vi "StatIntialse.vi"(0 "Init cluster 2":T1, 1 "Set Stability":T2(ring)=enum."Standard", 2 "Default\n Filter":T3(ring)=enum."10 kHz", 3 "error in (no error)":errorcluster, 4 "Default\nCurrent range":T4(ring)=enum."10 mA") -> (7 "Init cluster":T1, 10 "error out":errorcluster)   [LabVIEW 2020]
uses:
  Labview/IVIUM/IVIUM_remdriver.lvlib
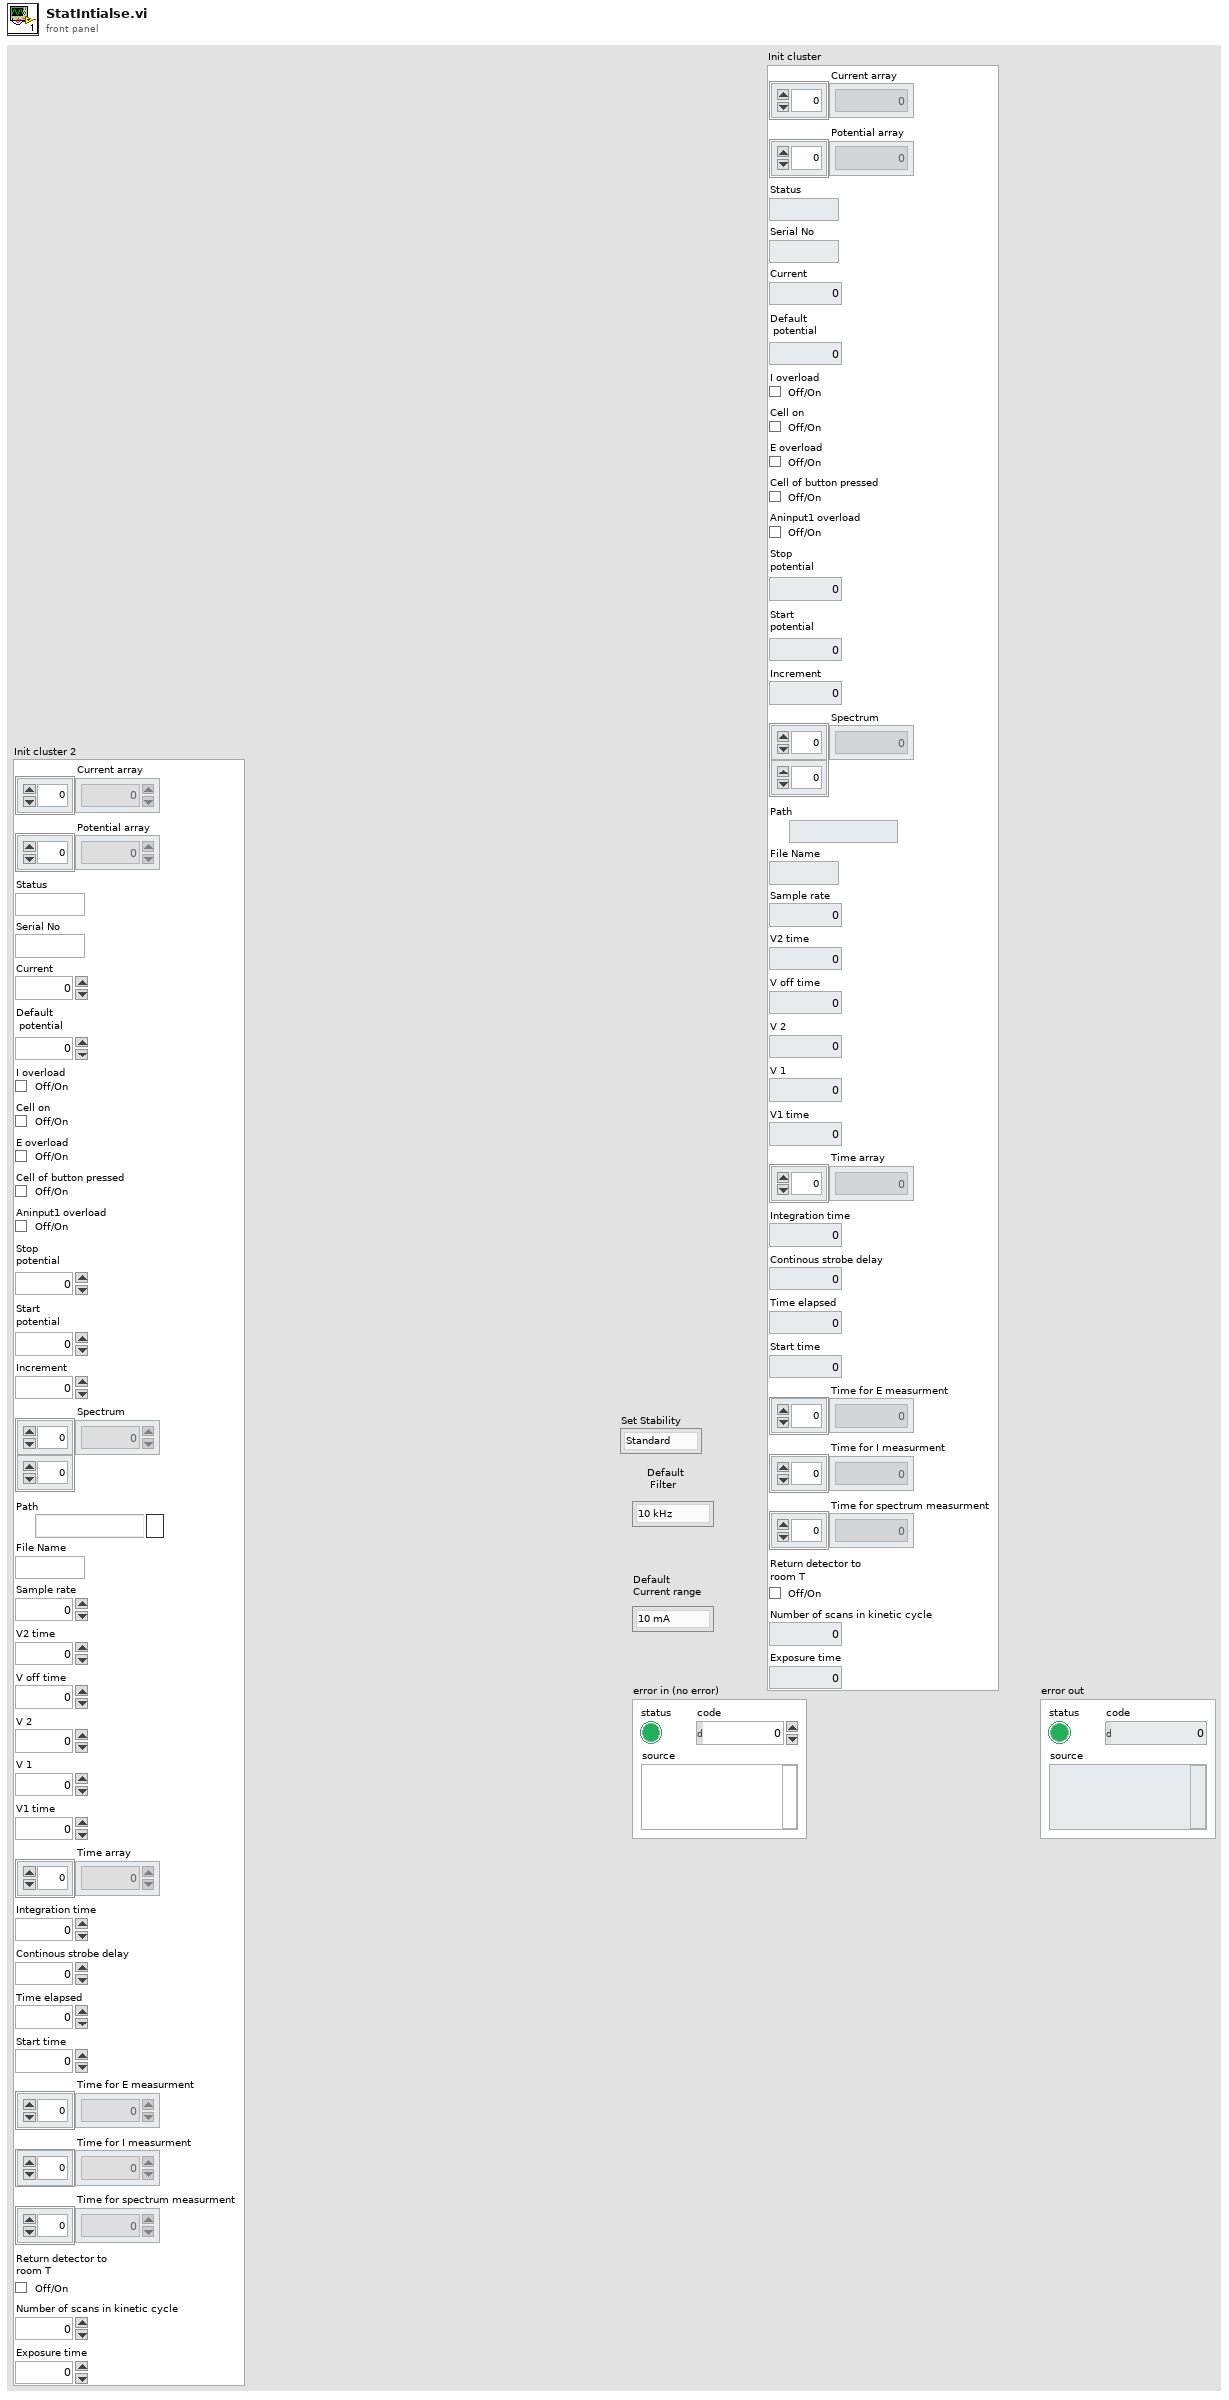
[diagram p1: front panel]
types:
  T1 = cluster{"Current array":dbl[], "Potential array":dbl[], "Status":string, "Serial No":string, "Current":dbl, "Default\n potential":dbl, "I overload":bool, "Cell on":bool, "E overload":bool, "Cell of button pressed":bool, "Aninput1 overload":bool, "Stop \npotential":dbl, "Start \npotential":dbl, "Increment":dbl, "Spectrum":dbl[][], "Path":path, "File Name":string, "Sample rate":dbl, "V2 time":dbl, "V off time":dbl, "V 2":dbl, "V 1":dbl, "V1 time":dbl, "Time array":dbl[], "Integration time":i32, "Continous strobe delay":i32, "Time elapsed ":i32, "Start time":i32, "Time for E measurment":i32[], "Time for I measurment ":i32[], "Time for spectrum measurment":i32[], "Return detector to \nroom T":bool, "Number of scans in kinetic cycle":i32, "Exposure time":i32}
  T2 = enum16{"High Speed", "Standard", "High Stability"}
  T3 = enum16{"1 MHz", "100 kHz", "10 kHz", "1 kHz", "10 Hz"}
  T4 = enum16{"10 A", "1 A", "100 mA", "10 mA", "1 mA", "100 uA", "10 uA", "1 uA", "100 nA", "10 nA", "1 nA", "100 pA", "10 pA", "1 pA"}
  T5 = enum16{"off", "EStat4EL", "EStat2EL", "EStatDummy1", "EStatDummy2", "EStatDummy3", "EStatDummy4", "IStat4EL", "IStat2EL", "IStatDummy", "BiStat4EL", "BiStat2EL"}
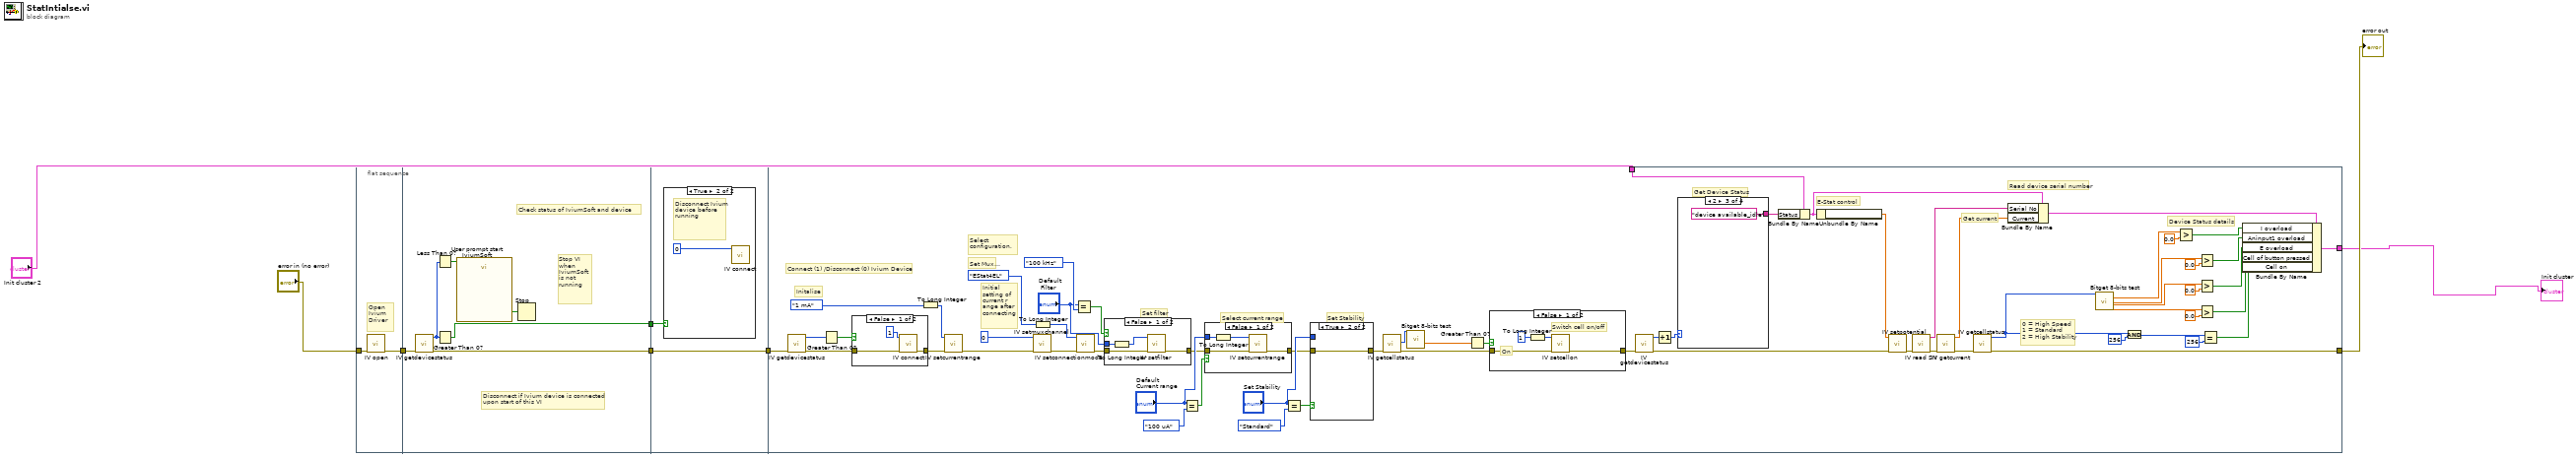
[diagram p0: block diagram]
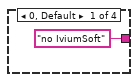
[diagram p5: hidden frame]
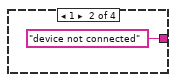
[diagram p6: hidden frame]
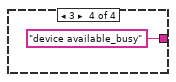
[diagram p7: hidden frame]
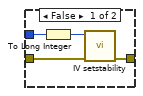
[diagram p8: hidden frame]
diagram:
  n1 = flat-sequence {
    tunnel: [w10] -> w7
    tunnel: "error in (no error)" -> [w9]
    tunnel: w7 -> [w13]
    tunnel: [w12] -> w5
    tunnel: [w11] -> w3
    tunnel: w5 -> [w18]
    tunnel: [w18] -> w4
    tunnel: w3 -> [w17]
    tunnel: "Init cluster 2" -> [w31]
    tunnel: [w45] -> w8
    tunnel: w4 -> [w22]
    tunnel: [w20] -> w1
    frame #0 {
      # "Open Ivium Driver"
      n2 = call "IV open.vi"("error in (no error)"=w9) -> ("error out"=w10:errorcluster)  [unwired: 9 in, 1 out]
    }
    frame #1 {
      # "Check status of IviumSoft and device"
      # "Stop VI when IviumSoft is not running"
      # "Disconnect if Ivium device is connected \nupon start of this VI"
      n3 = call "IV getdevicestatus.vi"("error in (no error)"=w13) -> ("error out"=w12:errorcluster, "return type"=w16:i32)  [unwired: 9 in]
      n4 = Less Than 0?(x=w16) -> (x < 0?=w14:bool)
      n5 = Greater Than 0?(x=w16) -> (x > 0?=w11:bool)
      n6 = call "User prompt start IviumSoft.vi"("Enable"=w14) -> ("OK"=w15:bool)  [unwired: 17 in, 1 out]
      n7 = Stop(stop? (T)=w15) -> ()
    }
    frame #2 {
      n8 = case shown="True" w17 {
        frame False {
        }
        frame True {
          # "Disconnect Ivium device before running"
          n9 = call "IV connect.vi"("devconnect"=0) -> ()  [unwired: 8 in, 3 out]
        }
      }
    }
    frame #3 {
      # "Device Status details"
      # "Get current"
      # "Set Mux channel"
      # "0 = High Speed\n1 = Standard \n2 = High Stability"
      # "Set Stability"
      # "Set filter"
      # "E-Stat control"
      # "Get Device Status"
      # "Select current range"
      # "Select configuration,"
      # "Read device serial number"
      # "Initial setting of current r\nange after connecting"
      # "Connect (1) /Disconnect (0) Ivium Device"
      # "Initalise"
      n10 = call "IV getdevicestatus.vi"("error in (no error)"=w22) -> ("error out"=w42:errorcluster, "return type"=w44:i32)  [unwired: 9 in]
      n11 = Greater Than 0?(x=w44) -> (x > 0?=w43:bool)
      n12 = case shown="False" w43 {
        tunnel: [w84 w85] -> w41
        tunnel: w42 -> [w82 w85]
        frame False {
          n13 = call "IV connect.vi"("error in (no error)"=w82, "devconnect"=1) -> ("error out"=w84:errorcluster)  [unwired: 7 in, 2 out]
        }
        frame True {
        }
      }
      n14 = To Long Integer(number=T4."1 mA" ("Current range selector")) -> (32bit integer=w40:i32)
      n15 = call "IV setcurrentrange.vi"("error in (no error)"=w41, "value"=w40) -> ("error out"=w39:errorcluster)  [unwired: 7 in, 2 out]
      n16 = call "IV setmuxchannel.vi"("error in (no error)"=w39, "value"=0) -> ("error out"=w38:errorcluster)  [unwired: 7 in, 2 out]
      n17 = To Long Integer(number=T5."EStat4EL" ("Configuration")) -> (32bit integer=w37:i32)
      n18 = Equal?(x="Default\n Filter", y=T3."100 kHz" ("Set Filter")) -> (x = y?=w75:bool)
      n19 = call "IV setconnectionmode.vi"("error in (no error)"=w38, "value"=w37) -> ("error out"=w35:errorcluster)  [unwired: 7 in, 2 out]
      n20 = case shown="False" w75 {
        tunnel: "Default\n Filter" -> [w103 _]
        tunnel: [w101 w104] -> w36
        tunnel: w35 -> [w100 w104]
        frame False {
          n21 = To Long Integer(number=w103) -> (32bit integer=w102:i32)
          n22 = call "IV setfilter.vi"("error in (no error)"=w100, "value"=w102) -> ("error out"=w101:errorcluster)  [unwired: 7 in, 2 out]
        }
        frame True {
        }
      }
      n23 = Equal?(x="Default\nCurrent range", y=T4."100 uA") -> (x = y?=w79:bool)
      n24 = case shown="False" w79 {
        tunnel: "Default\nCurrent range" -> [w107 _]
        tunnel: [w106 w109] -> w34
        tunnel: w36 -> [w105 w109]
        frame False {
          n25 = To Long Integer(number=w107) -> (32bit integer=w108:i32)
          n26 = call "IV setcurrentrange.vi"("error in (no error)"=w105, "value"=w108) -> ("error out"=w106:errorcluster)  [unwired: 7 in, 2 out]
        }
        frame True {
        }
      }
      n27 = Equal?(x="Set Stability", y=T2."Standard" ("Set Stability")) -> (x = y?=w77:bool)
      n28 = case shown="True" w77 {
        tunnel: "Set Stability" -> [w98 _]
        tunnel: [w96 w99] -> w33
        tunnel: w34 -> [w95 w99]
        frame False {
          n29 = To Long Integer(number=w98) -> (32bit integer=w97:i32)
          n30 = call "IV setstability.vi"("error in (no error)"=w95, "value"=w97) -> ("error out"=w96:errorcluster)  [unwired: 7 in, 2 out]
        }
        frame True {
        }
      }
      n31 = call "IV getcellstatus.vi"("error in (no error)"=w33) -> ("error out"=w47:errorcluster, "return type"=w51:i32)  [unwired: 8 in, 1 out]
      n32 = call "Bitget 8-bits test.vi"("x"=w51) -> ("f"=w50:dbl)  [unwired: 19 in, 7 out]
      n33 = Greater Than 0?(x=w50) -> (x > 0?=w49:bool)
      n34 = case shown="False" w49 {
        tunnel: w47 -> [w87 w90]
        tunnel: [w86 w90] -> w32
        frame False {
          # "On"
          # "Switch cell on/off"
          n35 = To Long Integer(number=1) -> (32bit integer=w89:i32)
          n36 = call "IV setcellon.vi"("error in (no error)"=w87, "cellon"=w89) -> ("error out"=w86:errorcluster)  [unwired: 7 in, 2 out]
        }
        frame True {
          # "If the cell is already\n on do nothing here"
        }
      }
      n37 = call "IV getdevicestatus.vi"("error in (no error)"=w32) -> ("error out"=w27:errorcluster, "return type"=w72:i32)  [unwired: 9 in]
      n38 = Increment(x=w72) -> (x+1=w71:i32)
      n39 = case shown="2" w71 {
        tunnel: ["no IviumSoft" "device not connected" "device available_idle" "device available_busy"] -> w57
        frame 0, Default {
        }
        frame 1 {
        }
        frame 2 {
        }
        frame 3 {
        }
      }
      n40 = Bundle By Name(cluster=w31, "Status"=w57) -> (w28:T1)
      n41 = Unbundle By Name(w28) -> ("Default\n potential"=w30:dbl)
      n42 = call "IV setpotential.vi"("error in (no error)"=w27, "value"=w30) -> ("error out"=w29:errorcluster)  [unwired: 7 in, 2 out]
      n43 = call "IV read SN.vi"("error in (no error)"=w29) -> ("error out"=w26:errorcluster, "sntext out"=w56:string)  [unwired: 8 in, 1 out]
      n44 = call "IV getcurrent.vi"("error in (no error)"=w26) -> ("error out"=w23:errorcluster, "value out"=w25:dbl)  [unwired: 8 in, 1 out]
      n45 = call "IV getcellstatus.vi"("error in (no error)"=w23) -> ("error out"=w45:errorcluster, "devcellstatus out"=w62:i32)  [unwired: 8 in, 1 out]
      n46 = Bundle By Name(cluster=w28, "Serial No"=w56, "Current"=w25) -> (w24:T1)
      n47 = call "Bitget 8-bits test.vi"("x"=w62) -> ("c"=w66:dbl, "e"=w64:dbl, "f"=w65:dbl, "h"=w63:dbl)  [unwired: 19 in, 4 out]
      n48 = And(x=w62, y=256) -> (x .and. y?=w60:i32)
      n49 = Greater?(x=w66, y=0.0) -> (0:w55:bool)
      n50 = Greater?(x=w64, y=0.0) -> (0:w54:bool)
      n51 = Greater?(x=w65, y=0.0) -> (0:w53:bool)
      n52 = Greater?(x=w63, y=0.0) -> (0:w21:bool)
      n53 = Equal?(x=w60, y=256) -> (x = y?=w52:bool)
      n54 = Bundle By Name(cluster=w24, "I overload"=w55, "Aninput1 overload"=w54, "E overload"=w53, "Cell of button pressed"=w21, "Cell on"=w52) -> (w20:T1)
    }
  }
  "error out" <- w8
  "Init cluster" <- w1
